vi "PH_Cam_BaseClass.Set Scroll Bars 2 Image.vi"(0 "i ref in":refnum<vi>, 5 "error in (no error)":errorcluster) -> (14 "i ref out":refnum<vi>, 19 "error out":errorcluster)   [LabVIEW 2014, in "PH_Cam_BaseClass.lvlib"]
doc: "This VI sets scroll bars to the image if the screen dimension is smaller than the image."
uses:
  PH_Cam_BaseClass.lvlib
  PH_StatusHandler/PH_StatusHandler.Status.ctl
  PH_StatusHandler/PH_StatusHandler.lvlib
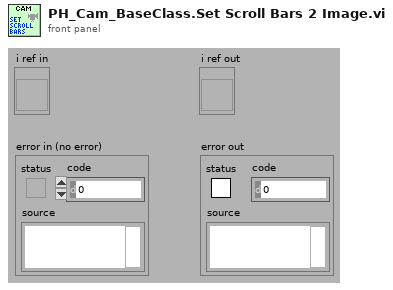
[diagram p1: front panel]
types:
  T1 = typedef "PH_StatusHandler.lvlib/PH_StatusHandler.Status.ctl" = i16
  T2 = typedef "PH_Cam_BaseClass.lvlib/PH_Cam_BaseClass.i attribute.ctl" = cluster{"Gui Refs":T3, "Cam":cluster{"Source Notifier":refnum<notifier>, "Error":errorcluster, "Camera ID":string}, "Images":cluster{"Cam":T4, "Operation":T4, "PSDB":T4}, "Window Image":cluster{"Indicate Image":bool, "Window No.":i32, "Scale Facor":dbl, "Center Cross":bool, "Subtract Backgr":bool, "CoG":bool, "Color Palette":cluster{"Red":u8, "Green":u8, "Blue":u8}[], "Image On":bool}, "Default Prdc Int":i32, "Performance":cluster{"on":bool, "Timestamp Last Frame":i32}, "Histogram":cluster{"on":bool, "Mapping":bool}, "Save Image":cluster{"Save":bool, "File refnum":refnum<file>}, "Setting Service ID":i32, "Screen":cluster{"x-resolution":i16, "y-resolution":i16}, "On":bool, "Constructor finished":bool, "configured":bool}
  T3 = typedef "PH_Cam_BaseClass.lvlib/PH_Cam_BaseClass.GUI Refs.ctl" = cluster{"Frame Rate":refnum<vi>, "Get Frame Rate":refnum<vi>, "Show Image":refnum<vi>, "Get Histogram":refnum<vi>, "Mapping":refnum<vi>, "Histogram":refnum<vi>, "Center Cross":refnum<vi>, "Center of Gravity":refnum<vi>, "Scale Factor [%]":refnum<vi>, "Save Image":refnum<vi>, "Palette":refnum<vi>, "Subtract Background":refnum<vi>, "Cam Error":refnum<vi>, "On":refnum<vi>, "Cam List":refnum<vi>}
  T4 = typedef "IMAQ Image.ctl" = refnum<image>
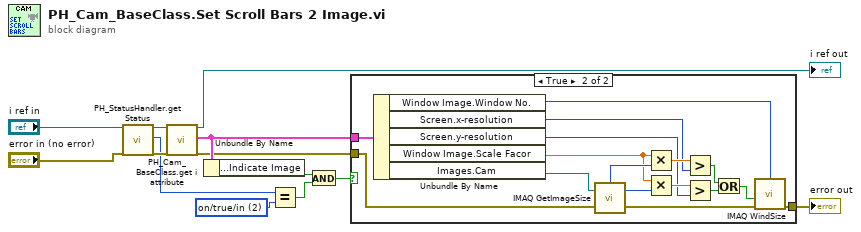
[diagram p0: block diagram]
diagram:
  w6 = T1 2 items=["no info", "off/false/out", "on/true/in", "Failure", "Alarm", "Status 1", "Status 2", "Status 3"] ("y")
  n1 = call "PH_StatusHandler.get Status.vi"("VI in"="i ref in", "error in"="error in (no error)") -> ("VI out"=w2:refnum<vi>, "Status"=w1:T1, "error out"=w4:errorcluster)  [unwired: 15 in]
  n2 = call "PH_Cam_BaseClass.get i attribute.vi"("i ref in"=w2, "error in (no error)"=w4) -> ("i ref out"=→"i ref out":refnum<vi>, "i attribute"=w13:T2, "error out"=w11:errorcluster)  [unwired: 15 in]
  n3 = Unbundle By Name(w13) -> ("Window Image.Indicate Image"=w9:bool)
  n4 = Equal?(x=w1, y=w6) -> (x = y?=w5:bool)
  n5 = And(x=w9, y=w5) -> (x .and. y?=w8:bool)
  n6 = case shown="True" w8 {
    tunnel: w13 -> [_ w27]
    tunnel: [w14 w18] -> w12
    tunnel: w11 -> [w14 w17]
    frame False {
    }
    frame True {
      n7 = Unbundle By Name(w27) -> ("Window Image.Window No."=w26:i32, "Screen.x-resolution"=w24:i16, "Screen.y-resolution"=w22:i16, "Window Image.Scale Facor"=w28:dbl, "Images.Cam"=w15:T4)
      n8 = call "IMAQ GetImageSize"("Image"=w15, "error in (no error)"=w17) -> ("Y Resolution"=w29:i32, "X Resolution"=w30:i32, "error out"=w16:errorcluster)  [unwired: 2 in]
      n9 = Multiply(x=w28, y=w30) -> (x*y=w25:dbl)
      n10 = Multiply(x=w28, y=w29) -> (x*y=w23:dbl)
      n11 = Greater?(x=w25, y=w24) -> (0:w21:bool)
      n12 = Greater?(x=w23, y=w22) -> (0:w20:bool)
      n13 = Or(x=w21, y=w20) -> (x .or. y?=w19:bool)
      n14 = call "IMAQ WindSize"("error in (no error)"=w16, "Scrollbars? (N)"=w19, "Window Number"=w26) -> ("error out"=w18:errorcluster)  [unwired: 3 in, 2 out]
    }
  }
  "error out" <- w12
